vi "checkCycleComplete.vi"(8 "error in (no error)":errorcluster, 11 "Model in":refnum<class "Model.lvclass">) -> (0 "error out":errorcluster, 2 "cycleCompleteIsTrue":bool, 3 "Model out":refnum<class "Model.lvclass">)   [LabVIEW 2015]
uses:
  ApplicationElements/TestMonitor/TestMonitor.lvclass
  Model.lvclass
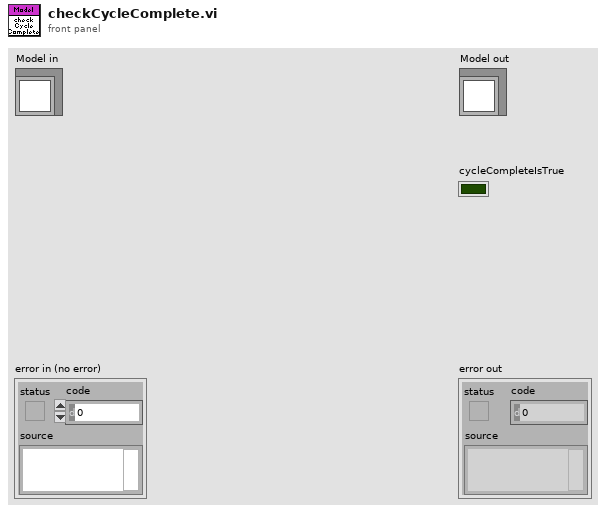
[diagram p1: front panel]
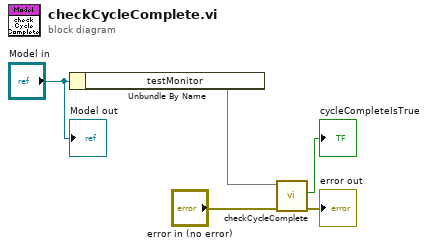
[diagram p0: block diagram]
diagram:
  n1 = Unbundle By Name("Model in") -> ("testMonitor"=w5)
  n2 = call "checkCycleComplete.vi"("error in (no error)"="error in (no error)", "TestMonitor in"=w5) -> ("error out"=→"error out":errorcluster, "cycleCompleteIsTrue"=→"cycleCompleteIsTrue":bool)  [unwired: 7 in, 1 out]
  "Model out" <- "Model in"
